vi "test_ccd_cleanCount.vi"(8 "error in":errorcluster, 11 "CCD in":refnum<class "CCD.lvclass">) -> (0 "error out":errorcluster, 3 "CCD out":refnum<class "CCD.lvclass">)   [LabVIEW 2020, in "horiba.test.lvlib"]
uses:
  horiba.test.lvlib
  Classes/CCD/CCD.lvclass
  <vilib>/addons/_JKI Toolkits/Caraya/classes/Assert/Assert Equal Value and Type_Variant.vi
  15e7fe39-3d4f-4ccc-ae5c-22e5f2c5c50b.vi
panel:
  # "Connector Pane"
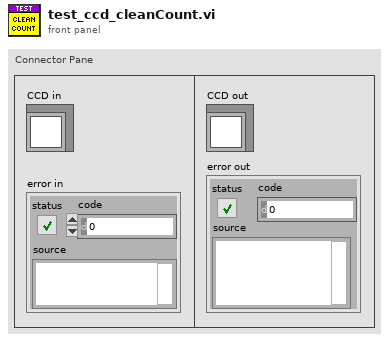
[diagram p1: front panel]
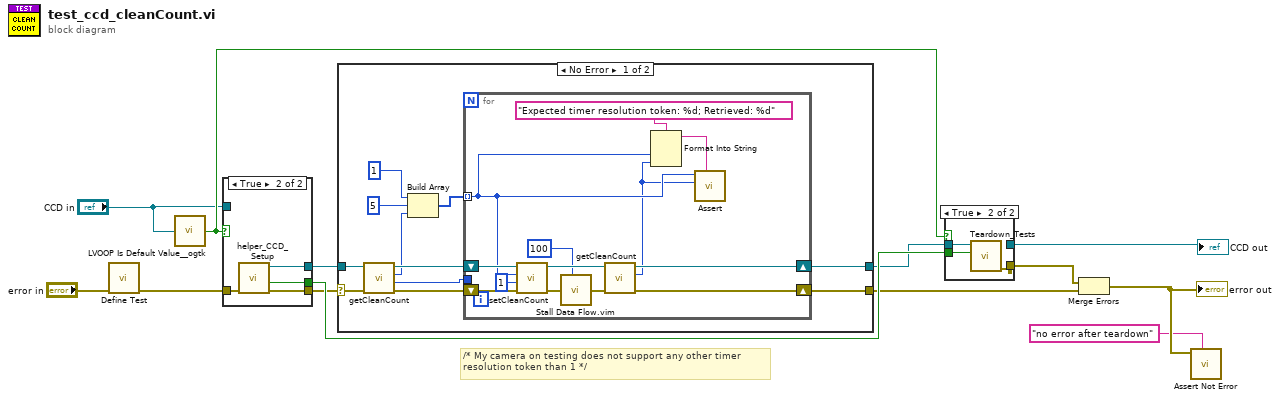
[diagram p0: block diagram]
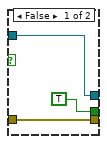
[diagram p3: hidden frame]
diagram:
  # "/* My camera on testing does not support any other timer \nresolution token than 1 */"
  n1 = call <vilib>:"Define Test.vi"("error in (no error)"="error in") -> ("error out"=w8:errorcluster)  [unwired: 9 in, 1 out]
  n2 = call <userlib>:"LVOOP Is Default Value__ogtk.vi"("Object"="CCD in") -> ("Is Default Value?"=w9:bool)
  n3 = case shown="True" w9 {
    tunnel: w8 -> [w15 w20]
    tunnel: [w15 w19] -> w4
    tunnel: [w16 w18] -> w6
    tunnel: [TRUE ("Module Was Already Running?") w17] -> w10
    tunnel: "CCD in" -> [w16 _]
    frame False {
    }
    frame True {
      n4 = call "helper_CCD_Setup.vi"("error in"=w20) -> ("error out"=w19:errorcluster, "Module Was Already Running?"=w17:bool, "CCD out"=w18:refnum<class "CCD.lvclass">)  [unwired: 7 in, 1 out]
    }
  }
  n5 = case shown="No Error" w4 {
    selector: w4 -> [w31 w45]
    tunnel: [w28 w46] -> w5
    tunnel: w6 -> [w30 w46]
    tunnel: [w26 w45] -> w3
    frame No Error {
      n6 = call "getCleanCount.vi"("error in (no error)"=w31, "CCD in"=w30) -> ("error out"=w27:errorcluster, "mode"=w21:i32, "count"=w22:i32, "CCD out"=w29:refnum<class "CCD.lvclass">)  [unwired: 6 in]
      n7 = Build Array(1 ("token"), 5 ("element"), w22) -> (w24:i32[])
      n8 = for {
        shift-right: [w41] -> w28
        shift-left: w29 -> [w42]
        shift-right: [w39] -> w26
        shift-left: w27 -> [w40]
        tunnel: w24 -> [w36] mode=indexing
        tunnel: w21 -> [_]
        n9 = call "setCleanCount.vi"("error in (no error)"=w40, "mode"=1, "count"=w36, "CCD in"=w42) -> ("error out"=w44:errorcluster, "CCD out"=w43:refnum<class "CCD.lvclass">)  [unwired: 4 in, 2 out]
        n10 = call "Stall Data Flow.vim"("value in"=w44, "milliseconds to wait"=u32 100) -> ("value out"=w34:errorcluster)  [unwired: 1 out]
        n11 = call "getCleanCount.vi"("error in (no error)"=w34, "CCD in"=w43) -> ("error out"=w39:errorcluster, "count"=w35:i32, "CCD out"=w41:refnum<class "CCD.lvclass">)  [unwired: 6 in, 1 out]
        n12 = Format Into String(format string="Expected timer resolution token: %d; Retrieved: %d", w36, w35) -> (resulting string=w38:string)  [unwired: 2 in, 1 out]
        n13 = call-poly <vilib>:"Assert.vi"("Label"=w38, "Y"=w35, "X"=w36) -> ()  [unwired: 7 in, 2 out]
      }
    }
    frame Error {
    }
  }
  n14 = case shown="True" w9 {
    tunnel: w5 -> [w47 w50]
    tunnel: [_ w49] -> w7
    tunnel: w10 -> [_ w48]
    tunnel: [w47 _] -> w1
    frame False {
    }
    frame True {
      n15 = call "Teardown_Tests.vi"("Module Was Already Running?"=w48, "horiba.lvlib:GenericDevice"=w50) -> ("error out"=w49:errorcluster)  [unwired: 8 in, 1 out]
    }
  }
  "CCD out" <- w1
  n16 = Merge Errors(w7, w3) -> (w12:errorcluster)
  "error out" <- w12
  n17 = call <vilib>:"Assert Not Error.vi"("Label"="no error after teardown", "Not Error?"=w12) -> ()  [unwired: 8 in, 2 out]
